vi "Filter Aliases from Connection List.vi"(8 "error in (no error)":errorcluster, 10 "Alias Mapping":T1, 11 "Connection List in":T2[](array[typedef])) -> (0 "error out":errorcluster, 3 "Connection List out":T2[](array[typedef]))   [LabVIEW 2017, in "Routing and Faulting System Explorer.lvlib"]
uses:
  Routing and Faulting System Explorer.lvlib
  Shared/Connection.ctl
  Shared/Alias Mapping.ctl
  Shared/Routing and Faulting Shared.lvlib
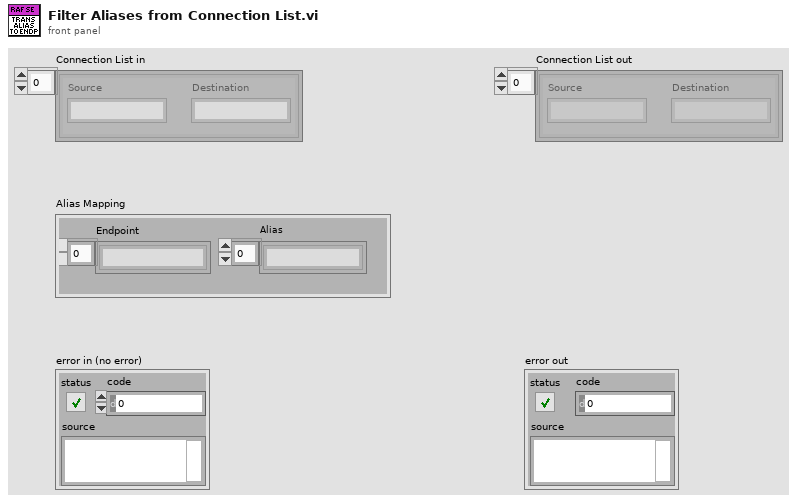
[diagram p1: front panel]
types:
  T1 = typedef "Routing and Faulting Shared.lvlib/Alias Mapping.ctl" = cluster{"Endpoint":string[], "Alias":string[]}
  T2 = typedef "Routing and Faulting Shared.lvlib/Connection.ctl" = cluster{"Source":string, "Destination":string}
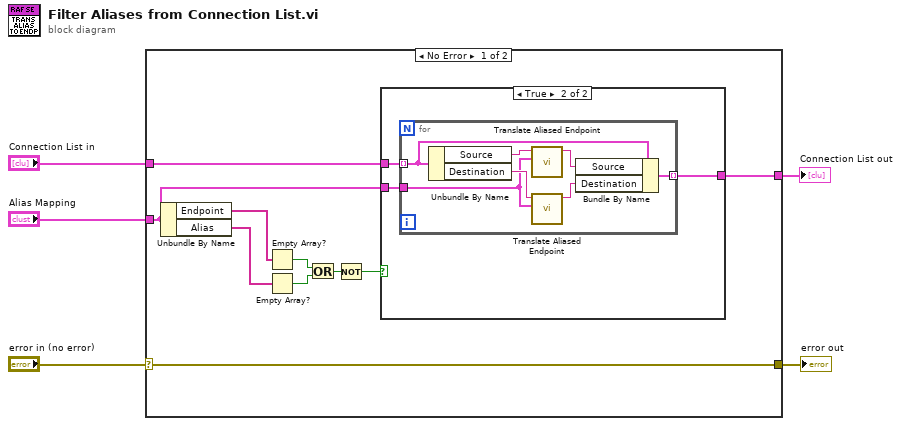
[diagram p0: block diagram]
diagram:
  n1 = case shown="No Error" "error in (no error)" {
    selector: "error in (no error)" -> [w14 w28]
    tunnel: "Connection List in" -> [w15 w27]
    tunnel: [w14 w28] -> w3
    tunnel: "Alias Mapping" -> [w6 _]
    tunnel: [w9 w27] -> w1
    frame No Error {
      n2 = Unbundle By Name(w6) -> ("Endpoint"=w7:string[], "Alias"=w8:string[])
      n3 = Empty Array?(array=w7) -> (empty?=w13:bool)
      n4 = Empty Array?(array=w8) -> (empty?=w12:bool)
      n5 = Or(x=w13, y=w12) -> (x .or. y?=w11:bool)
      n6 = Not(x=w11) -> (.not. x?=w10:bool)
      n7 = case shown="True" w10 {
        tunnel: w15 -> [w16 w19]
        tunnel: [w16 w17] -> w9
        tunnel: w6 -> [_ w18]
        frame False {
        }
        frame True {
          n8 = for {
            tunnel: w19 -> [w23] mode=indexing
            tunnel: w18 -> [w24]
            tunnel: [w20] -> w17 mode=indexing
            n9 = Unbundle By Name(w23) -> ("Source"=w26:string, "Destination"=w25:string)
            n10 = call "Translate Aliased Endpoint.vi"("Alias Mapping"=w24, "Endpoint in"=w26) -> ("Endpoint out"=w22:string)  [unwired: 9 in]
            n11 = call "Translate Aliased Endpoint.vi"("Alias Mapping"=w24, "Endpoint in"=w25) -> ("Endpoint out"=w21:string)  [unwired: 9 in]
            n12 = Bundle By Name(cluster=w23, "Source"=w22, "Destination"=w21) -> (w20:T2)
          }
        }
      }
    }
    frame Error {
    }
  }
  "error out" <- w3
  "Connection List out" <- w1
